vi "Fail_List.vi"(8 "error in (no error)":errorcluster, 10 "Label.Text":string, 11 "Ref in":T1={"MS SQL Connection"=refnum, "UDL File"=path "", "Time"="", "DCODE"="", "WIP+1"=0, "MC No?"=0, "POKAYOKE?"=FALSE, "Expected Result"="", "Result [Status]"="", "Clock"=0.0, "RFID"="", "WIP Queue"=refnum, "TS Parameter"={"ProfitCenterCode"="", "LineCode"="", "WorkOrderNumber"="", "Model"="", "Model_with_Prefix"="", "VendorCode"="", "SetParameterDateCode"="", "PokaYoke"=0, "Target"=1, "Live_DateCode"="", "CustomerPartNumber"="", "Hand"="", "sBarcode"=FALSE, "FCA"=0, "Ent_Stamp"=timestamp(0 s since 1904-01-01), "STS_CD"=0.0}, "Data_Queue"=[], "RFID Serial No."=""} {"TS Parameter"."FCA" format="%01d"; "TS Parameter"."Target" min=1 max=100000; "TS Parameter"."PokaYoke" min=0 max=1}) -> (0 "error out":errorcluster)   [LabVIEW 2020]
uses:
  Controls/TD SQL.ctl
  <vilib>/addons/database/Connection.llb/Conn ObjectReference.ctl
  Controls/WIP_State.ctl
  Controls/TS_Parameter.ctl
  <vilib>/Utility/miscctls.llb/LVRowAndColumnTypeDef.ctl
  MS SQL/MS_Global.vi
  <vilib>/addons/database/NI_Database_API.lvlib
panel:
  in  "WIP List 2":i32(listbox)
  in  "Exit":bool
  in  "WIP List":i32(listbox)
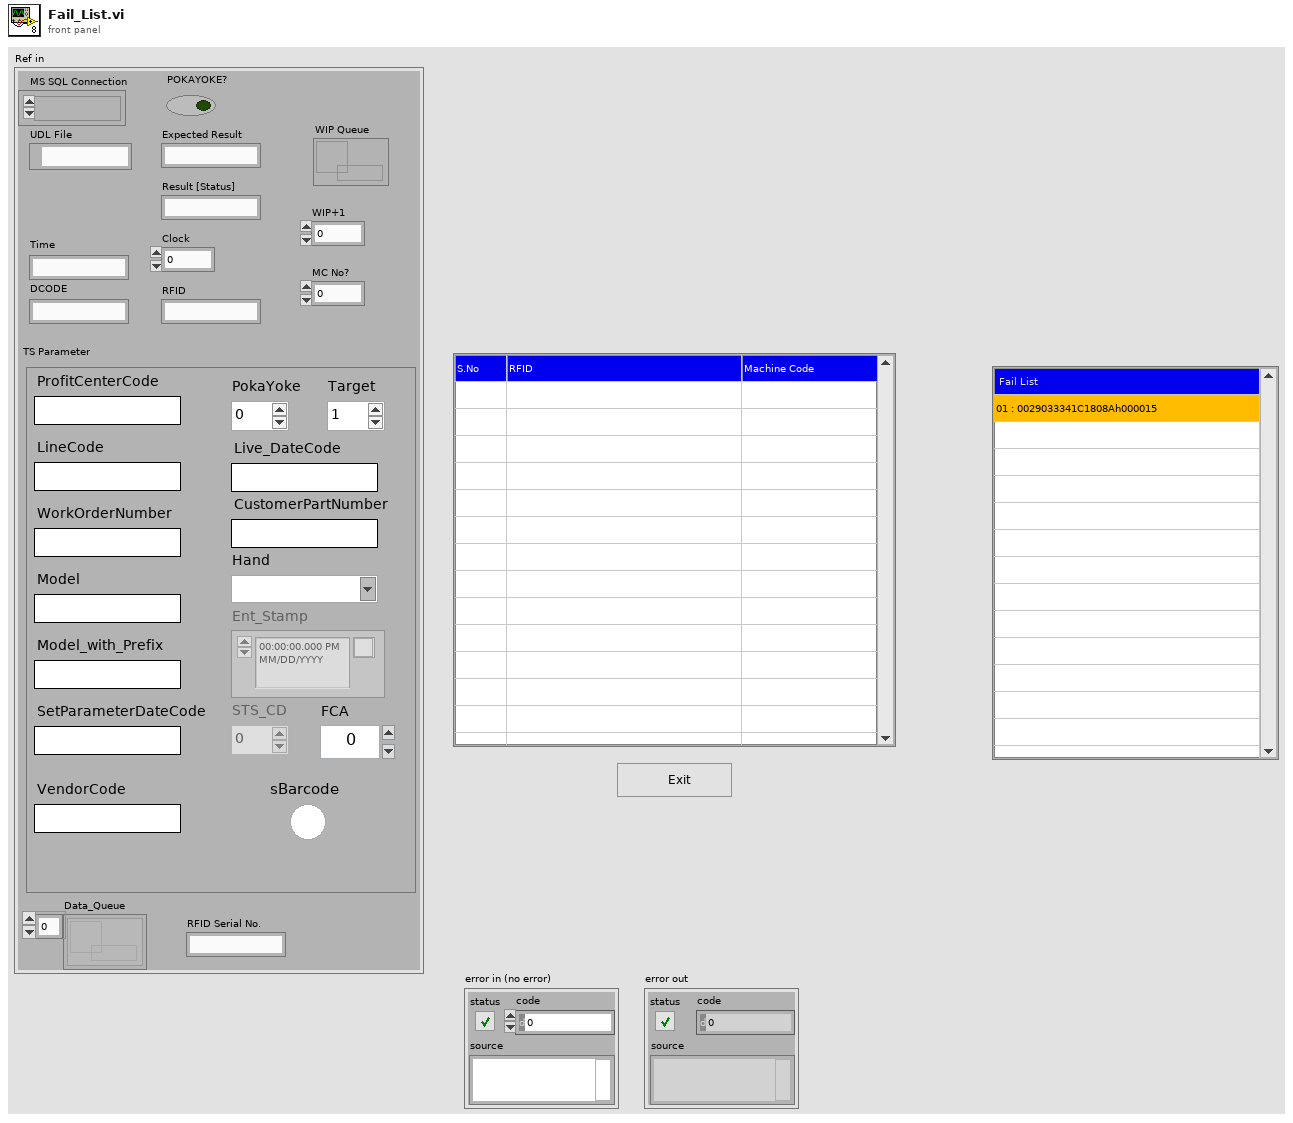
[diagram p1: front panel]
types:
  T1 = typedef "TD SQL.ctl" = cluster{"MS SQL Connection":T2, "UDL File":path, "Time":string, "DCODE":string, "WIP+1":i64, "MC No?":i32, "POKAYOKE?":bool, "Expected Result":string, "Result [Status]":string, "Clock":dbl, "RFID":string, "WIP Queue":refnum<queue>, "TS Parameter":T3, "Data_Queue":refnum<queue>[], "RFID Serial No.":string}
  T2 = typedef "NI_Database_API.lvlib/Conn ObjectReference.ctl" = refnum<k1>
  T3 = typedef "TS_Parameter.ctl" = cluster{"ProfitCenterCode":string, "LineCode":string, "WorkOrderNumber":string, "Model":string, "Model_with_Prefix":string, "VendorCode":string, "SetParameterDateCode":string, "PokaYoke":i32, "Target":i32, "Live_DateCode":string, "CustomerPartNumber":string, "Hand":string, "sBarcode":bool, "FCA":i32, "Ent_Stamp":timestamp, "STS_CD":dbl}
  T4 = typedef "LVRowAndColumnTypeDef.ctl" = cluster{"Row":i32, "Column":i32}
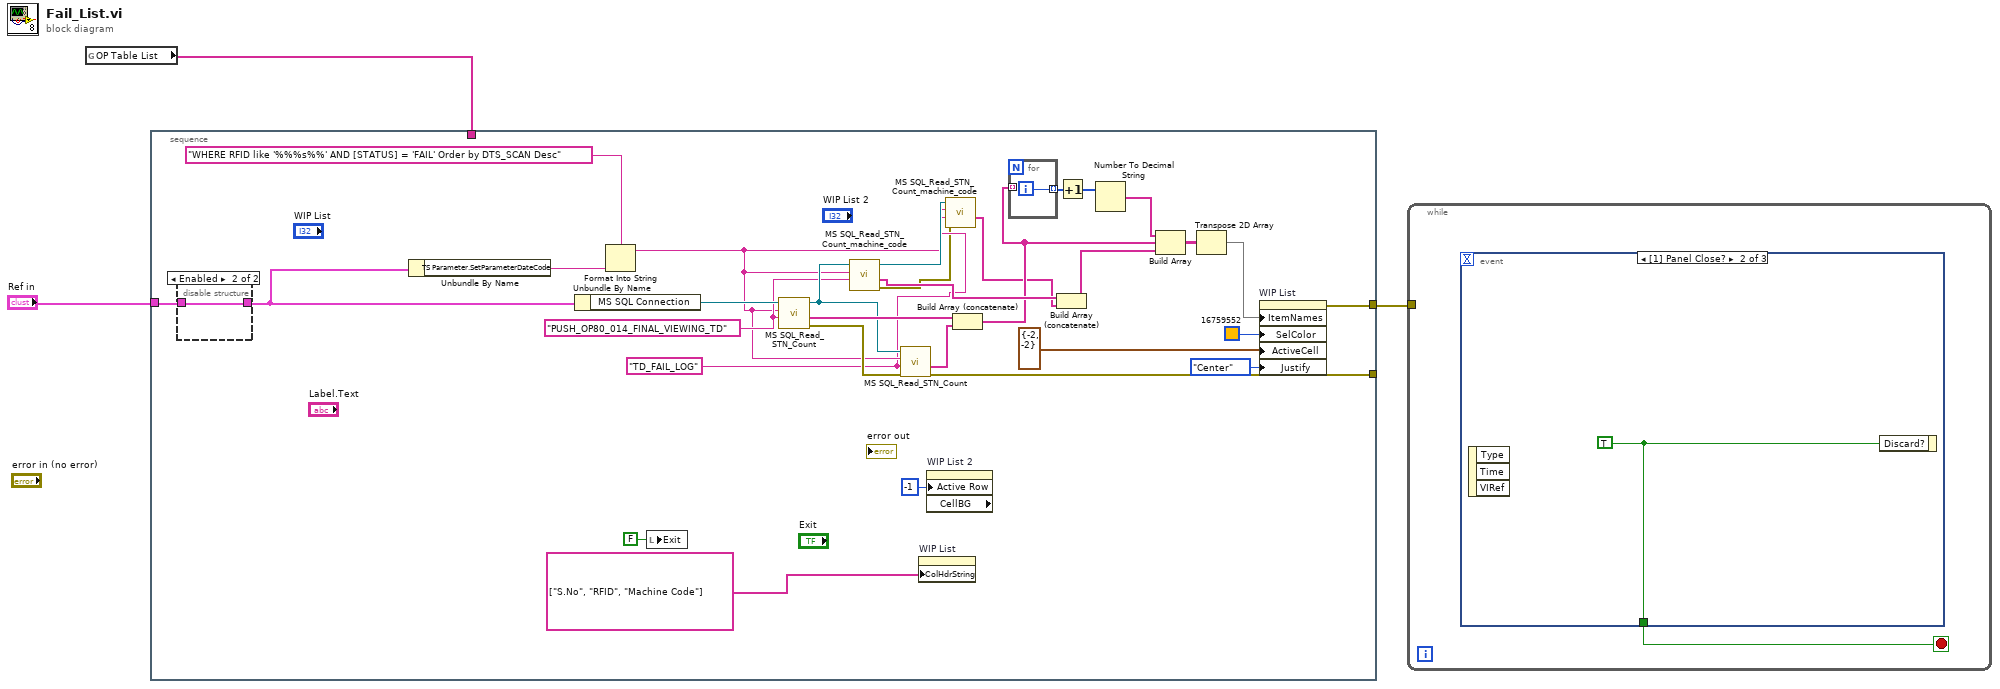
[diagram p0: block diagram]
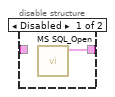
[diagram p2: hidden frame]
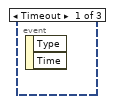
[diagram p3: hidden frame]
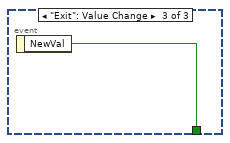
[diagram p4: hidden frame]
diagram:
  n1 = global read "MS_Global.vi" "OP Table List"() -> (w2:string[])
  n2 = stacked-sequence {
    tunnel: [w32] -> w3
    tunnel: w2 -> [_]
    tunnel: "Ref in" -> [w28]
    tunnel: [w26] -> _
    frame #0 {
      w9 = "TD_FAIL_LOG" ("Label.Text")
      w19 = "PUSH_OP80_014_FINAL_VIEWING_TD" ("Label.Text")
      n3 = disable-structure shown="Enabled" {
        disable-tunnel: w28 -> [_ w37]
        disable-tunnel: [w36 w37] -> w5
        frame Disabled {
          n4 = call "MS SQL_Open.vi"() -> ("Ref Out"=w36:T1)  [unwired: 9 in, 2 out]
        }
        frame Enabled {
        }
      }
      n5 = Unbundle By Name(w5) -> ("TS Parameter.SetParameterDateCode"=w4:string)
      n6 = Unbundle By Name(w5) -> ("MS SQL Connection"=w34:T2)
      n7 = Format Into String(format string="WHERE RFID like '%%%s%%' AND [STATUS] = 'FAIL' Order by DTS_SCAN Desc" ("Query"), w4) -> (resulting string=w10:string)  [unwired: 2 in, 1 out]
      n8 = local write "Exit"(FALSE ("Exit")) -> ()
      n9 = call "MS SQL_Read_STN_Count.vi"("Table?"=w19, "Query"=w10, "Refnum in"=w34) -> ("error out"=w21:errorcluster, "RFID"=w30:string[], "Refnum out"=w20:T2)  [unwired: 5 in, 1 out]
      n10 = call "MS SQL_Read_STN_Count_machine_code.vi"("Table?"=w19, "Query"=w10, "Refnum in"=w20) -> ("error out"=w7:errorcluster, "MACHINECODE"=w18:string[], "Refnum out"=w11:T2)  [unwired: 5 in, 1 out]
      n11 = call "MS SQL_Read_STN_Count.vi"("error in (no error)"=w21, "Table?"=w9, "Query"=w10, "Refnum in"=w20) -> ("error out"=w26:errorcluster, "RFID"=w27:string[])  [unwired: 4 in, 2 out]
      n12 = property on="WIP List" class="MCListbox (strict)"("ColHdrString"=string[] ["S.No", "RFID", "Machine Code"] ("Column Header Strings[]")) -> ()  [unwired: 2 in, 2 out]
      n13 = property on="WIP List 2" class="LstBox (strict)" props=["Active Row", "CellBG"]("Active Row"=-1 ("Active Row:Active Row Number")) -> ()  [unwired: 2 in, 3 out]
      n14 = call "MS SQL_Read_STN_Count_machine_code.vi"("error in (no error)"=w7, "Table?"=w9, "Query"=w10, "Refnum in"=w11) -> ("MACHINECODE"=w8:string[])  [unwired: 4 in, 3 out]
      n15 = Build Array (concatenate)(w30, w27) -> (w16:string[])
      n16 = for {
        tunnel: w16 -> [_] mode=indexing
        tunnel: [w35] -> w15 mode=indexing
        i -> [w35]
      }
      n17 = Build Array (concatenate)(w18, w8) -> (w17:string[])
      n18 = Increment(x=w15) -> (x+1=w13:i32[])
      n19 = Number To Decimal String(number=w13) -> (decimal integer string=w14:string[])  [unwired: 1 in]
      n20 = Build Array(w14, w16, w17) -> (w24:string[][])
      n21 = Transpose 2D Array(2D array=w24) -> (transposed array=w12:string[][])
      n22 = property on="WIP List" class="MCListbox (strict)"("ItemNames"=w12, "SelColor"=u32 16759552 ("Selection Color"), "ActiveCell"=T4 {"Row"=-2, "Column"=-2} ("Active Cell:Active Cell"), "Justify"=enum16{"Left", "Center", "Right"}."Center" ("Active Cell:Cell Justification")) -> (error out=w32:errorcluster)  [unwired: 2 in, 1 out]
    }
  }
  n23 = while {
    tunnel: w3 -> [_]
    stop <- w38 stop-if-true
    n24 = event shown="[1] Panel Close?" {
      selector: _ -> [_ _ _]
      dyn-events: _ -> [_ _ _]
      timeout: _ -> [_ _ _]
      tunnel: [_ w39 w40] -> w38
      event Timeout {
        n25 = event-data() -> ()  [unwired: 1 in, 2 out]
      }
      event Panel Close? {
        w39 = TRUE ("Discard?")
        n26 = event-data() -> ()  [unwired: 1 in, 3 out]
        n27 = event-data("Discard?"=w39) -> ()  [unwired: 1 in, 1 out]
      }
      event "Exit": Value Change {
        n28 = event-data() -> ("NewVal"=w40:bool)  [unwired: 1 in]
      }
    }
  }
